vi "LIDAR V2 Globals.vi"() -> ()   [LabVIEW 2015]
uses:
  Controls/Algorithm State.ctl
panel:
  in  "SubstractDark":bool
  in  "SampPerPulse":u32
  in  "MaxMem0":u32
  in  "MaxMem1":u32
  in  "MaxStartSample":u32
  in  "10thIndex":u8
  in  "10thIndex2":u8
  in  "10thIndex1":u8
  out "AlgoLedIndex":u8
  out "AlgoState":T1
  out "SimFineMaxIndex":u16
  out "SimCoarsMaxIndex":u16
  in  "Max 0":u32
  in  "Max 19":u32
  in  "Max 18":u32
  in  "Max 17":u32
  in  "Max 16":u32
  in  "Max 15":u32
  in  "Max 14":u32
  in  "Max 13":u32
  in  "Max 12":u32
  in  "Max 11":u32
  in  "Max 10":u32
  in  "Max 9":u32
  in  "Max 8":u32
  in  "Max 7":u32
  in  "Max 6":u32
  in  "Max 5":u32
  in  "Max 4":u32
  in  "Max 3":u32
  in  "Max 2":u32
  in  "Max 1":u32
  in  "ActiveLedIndex":u16
  in  "LastItteration":bool
  in  "SampEn":bool
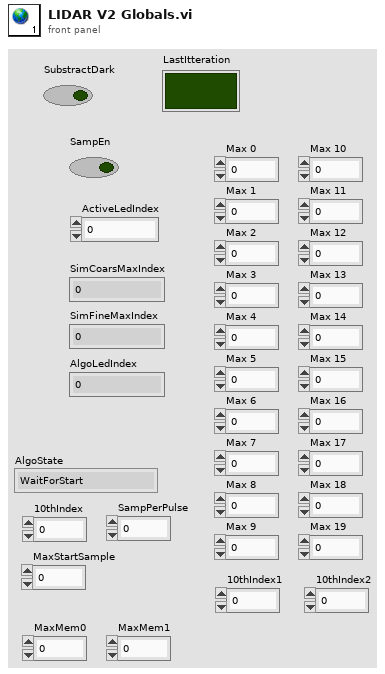
[diagram p1: front panel]
types:
  T1 = typedef "Algorithm State.ctl" = enum16{"WaitForStart", "GetNextSignalElement", "WaitForNextSignalElem", "MultWithSinc", "CalcMax"}
diagram:
